vi "4155C Transfer.vi"(0 "VISA resource name in":refnum<visa-resource-name>="GPIB0::14::INSTR", 2 "Gate":T5={"Gate Start"=0.0, "Gate Stop"=2.0, "Gate Step (linear only)"=1.0, "Gate Compliance"=0.0001, "Gate PComp"=0.0, "Range mode"=0, "Range"=6} {"Range" max=11 scale=0.0..11.0; "Range mode" items=["Auto", "Limited", "Fixed"]; "Gate PComp" min=0.0 max=2.0 format="%^.2e"; "Gate Compliance" min=0.0 max=0.1 format="%^.2e"; "Gate Step (linear only)" min=-100.0 max=100.0 format="%^.4e"; "Gate Stop" min=-100.0 max=100.0 format="%^.4e"; "Gate Start" min=-100.0 max=100.0 format="%^.4e"}, 3 "Drain":T6={"Drain Start"=0.0, "Drain Stop"=2.0, "Drain Compliance"=0.0001, "Drain Step"=1.0, "Drain PComp"=0.0, "Range mode"=0, "Range"=6} {"Range" max=11 scale=0.0..11.0; "Range mode" items=["Auto", "Limited", "Fixed"]; "Drain PComp" min=0.0 max=2.0 format="%^.2e"; "Drain Step" min=-100.0 max=100.0 format="%^.4e"; "Drain Compliance" min=0.0 max=0.1 format="%^.2e"; "Drain Stop" min=-100.0 max=100.0 format="%^.4e"; "Drain Start" min=-100.0 max=100.0 format="%^.4e"}, 5 "Timings":T4={"integration time"=0, "Short/Long integration time"=0.00064, "hold time (sec)"=0.0, "delay time (sec)"=0.0, "Step Time (0 disables)"=0.0, "sweep method"=0, "Pulse period"=0.005, "Base voltage"=0.0, "Pulse width"=0.0005} {"Pulse width" min=0.0005 max=0.1 step=0.0001 format="%.4f"; "Base voltage" min=-100.0 max=100.0 format="%^.4e"; "Pulse period" min=0.005 max=1.0 step=0.0001 format="%.4f"; "sweep method" items=["Continuous", "Pulsed"]; "Step Time (0 disables)" min=0.0 format="%.2f"; "delay time (sec)" min=0.0 format="%.4f"; "hold time (sec)" min=0.0 format="%.4f"; "Short/Long integration time" min=0.0 format="%^.0e"; "integration time" scale=0.0..2.0}, 6 "error in (no error)":errorcluster, 7 "SMU4":cluster{"on/off":bool, "Voltage":dbl} {"Voltage" min=-100.0 max=100.0 format="%.2f"}, 10 "sweep mode":u16(ring) items=["Single", "Double"], 12 "Panel Controls":T3={"Emergency Stop"=refnum, "TransGraph Max"=1e-05, "Text/Graph (text=false)"=FALSE, "TransGraph Min"=1e-11} {"TransGraph Min" format="%.2e"; "TransGraph Max" format="%.2e"}, 13 "Standby":T1) -> (16 "VG":dbl[](array[numeric]) format="%.2f", 17 "Outparams":T2={"V2 Start"=0.0, "V2 Step"=0.0, "Number of points"=1} {"V2 Step" format="%.2f"; "V2 Start" format="%^.4e"}, 20 "VISA Resource Name out":refnum<visa-resource-name>, 22 "IS":dbl[](array[numeric]) format="%.2f", 23 "ID":dbl[](array[numeric]) format="%.2f", 25 "IG":dbl[](array[numeric]) format="%.2f", 26 "error out":errorcluster, 27 "SMU4":dbl[](array[numeric]) format="%.2f")   [LabVIEW 2016]
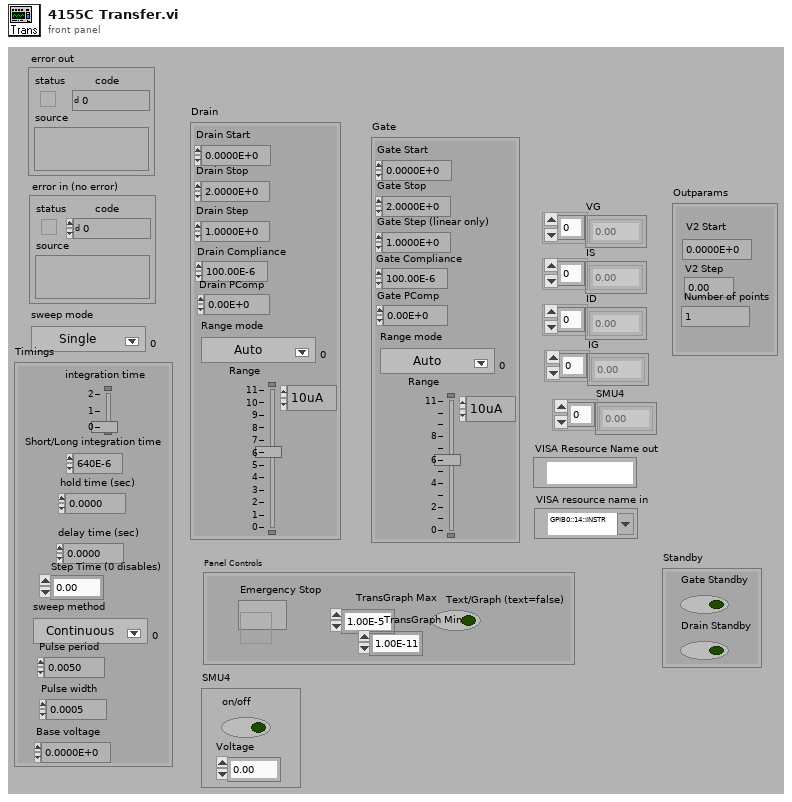
[diagram p1: front panel]
types:
  T1 = cluster{"Gate Standby":bool, "Drain Standby":bool}
  T2 = cluster{"V2 Start":dbl, "V2 Step":dbl, "Number of points":i32}
  T3 = cluster{"Emergency Stop":refnum<vi>, "TransGraph Max":dbl, "Text/Graph (text=false)":bool, "TransGraph Min":dbl}
  T4 = cluster{"integration time":u32, "Short/Long integration time":dbl, "hold time (sec)":dbl, "delay time (sec)":dbl, "Step Time (0 disables)":dbl, "sweep method":u16, "Pulse period":dbl, "Base voltage":dbl, "Pulse width":dbl}
  T5 = cluster{"Gate Start":dbl, "Gate Stop":dbl, "Gate Step (linear only)":dbl, "Gate Compliance":dbl, "Gate PComp":dbl, "Range mode":u16, "Range":u8}
  T6 = cluster{"Drain Start":dbl, "Drain Stop":dbl, "Drain Compliance":dbl, "Drain Step":dbl, "Drain PComp":dbl, "Range mode":u16, "Range":u8}
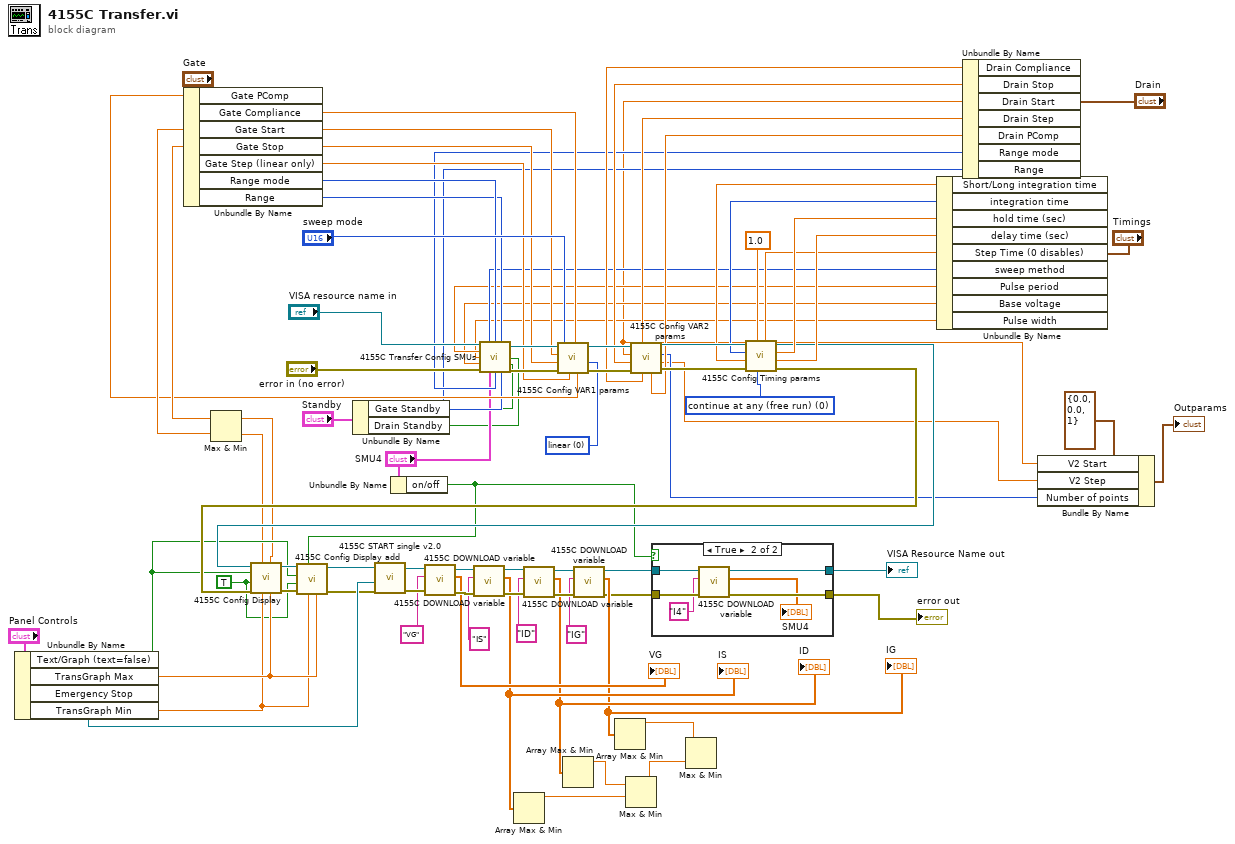
[diagram p0: block diagram]
diagram:
  w5 = TRUE ("Logarithmic")
  w69 = u8 0 items=["continue at any (free run)", "stop at any abnorm", "stop at compliance"] ("stop condition (free run:0)")
  w66 = u16 0 items=["linear", "log 10", "log 25", "log 50"] ("sweep spacing (linear: 0)")
  n1 = Unbundle By Name("Panel Controls") -> ("Text/Graph (text=false)"=w4:bool, "TransGraph Max"=w7:dbl, "Emergency Stop"=w36:refnum<vi>, "TransGraph Min"=w6:dbl)
  n2 = Unbundle By Name("Gate") -> ("Gate PComp"=w34:dbl, "Gate Compliance"=w55:dbl, "Gate Start"=w38:dbl, "Gate Stop"=w37:dbl, "Gate Step (linear only)"=w54:dbl, "Range mode"=w32:u16, "Range"=w31:u8)
  n3 = Max & Min(x=w37, y=w38) -> (max(x,y)=w1:dbl, min(x,y)=w2:dbl)
  n4 = Unbundle By Name("Standby") -> ("Gate Standby"=w13:bool, "Drain Standby"=w12:bool)
  n5 = Unbundle By Name("SMU4") -> ("on/off"=w3:bool)
  n6 = Unbundle By Name("Timings") -> ("Short/Long integration time"=w71:dbl, "integration time"=w49:u32, "hold time (sec)"=w50:dbl, "delay time (sec)"=w51:dbl, "Step Time (0 disables)"=w48:dbl, "sweep method"=w28:u16, "Pulse period"=w27:dbl, "Base voltage"=w25:dbl, "Pulse width"=w26:dbl)
  n7 = Unbundle By Name("Drain") -> ("Drain Compliance"=w58:dbl, "Drain Stop"=w57:dbl, "Drain Start"=w20:dbl, "Drain Step"=w56:dbl, "Drain PComp"=w33:dbl, "Range mode"=w30:u16, "Range"=w29:u8)
  n8 = call "4155C Transfer Config SMUs.vi"("VISA resource name in"="VISA resource name in", "sweep method"=w28, "Gate mode"=w32, "Gate Range"=w31, "Pulse period"=w27, "Pulse width"=w26, "Drain Standby"=w12, "Base voltage"=w25, "Gate Standby"=w13, "error in (no error)"="error in (no error)", "SMU4"="SMU4", "Source/drain mode"=w30, "Source/drain Range"=w29) -> ("VISA Resource Name out"=w64:refnum<visa-resource-name>, "error out"=w63:errorcluster)  [unwired: 1 in]
  n9 = call "4155C Config VAR1 params.vi"("sweep spacing (linear: 0)"=w66, "power compliance (0 = OFF)"=w34, "compliance"=w55, "step (linear only)"=w54, "sweep mode"="sweep mode", "error in (no error)"=w63, "stop"=w37, "start"=w38, "VISA session"=w64) -> ("error out"=w67:errorcluster, "dup VISA resource name"=w68:refnum<visa-resource-name>)  [unwired: 1 out]
  n10 = call "4155C Config VAR2 params.vi"("power compliance (0 = OFF)"=w33, "compliance"=w58, "step"=w56, "error in (no error)"=w67, "stop"=w57, "start"=w20, "VISA session"=w68) -> ("error out"=w72:errorcluster, "Corrected Step"=w21:dbl, "Number of points"=w22:i32, "dup VISA resource name"=w73:refnum<visa-resource-name>)  [unwired: 1 in]
  n11 = call "4155C Config Timing params.vi"("delay time (sec)"=w51, "hold time (sec)"=w50, "Step Time (0 disables)"=w48, "stop condition (free run:0)"=w69, "wait time parameter"=1.0, "error in (no error)"=w72, "Short/Long integration time"=w71, "integration time"=w49, "VISA session"=w73) -> ("error out"=w40:errorcluster, "dup VISA resource name"=w39:refnum<visa-resource-name>)  [unwired: 1 in]
  n12 = call "4155C Config Display.vi"("Ymax"=w7, "Var1 Stop"=w1, "Ymin"=w6, "Var1 Start"=w2, "error in (no error)"=w40, "Logarithmic"=w5, "SPA Display"=w4, "VISA session"=w39) -> ("error out"=w8:errorcluster, "dup VISA resource name"=w11:refnum<visa-resource-name>)  [unwired: 2 in]
  n13 = call "4155C Config Display add.vi"("Ymax"=w7, "Ymin"=w6, "SMU4"=w3, "error in (no error)"=w8, "Logarithmic"=w5, "SPA Display"=w4, "VISA session"=w11) -> ("error out"=w9:errorcluster, "dup VISA resource name"=w10:refnum<visa-resource-name>)  [unwired: 3 in]
  n14 = call "4155C START single v2.0.vi"("error in (no error)"=w9, "Emergency Stop"=w36, "VISA resource name in"=w10) -> ("error out"=w84:errorcluster, "VISA Resource Name out"=w85:refnum<visa-resource-name>)  [unwired: 3 in]
  n15 = call "4155C DOWNLOAD variable.vi"("error in (no error)"=w84, "Variable name"="VG", "VISA resource name in"=w85) -> ("error out"=w82:errorcluster, "Output data"=→"VG":dbl[], "VISA Resource Name out"=w81:refnum<visa-resource-name>)  [unwired: 2 in]
  n16 = call "4155C DOWNLOAD variable.vi"("error in (no error)"=w82, "Variable name"="IS", "VISA resource name in"=w81) -> ("error out"=w78:errorcluster, "Output data"=w47:dbl[], "VISA Resource Name out"=w79:refnum<visa-resource-name>)  [unwired: 2 in]
  "IS" <- w47
  n17 = Array Max & Min(array=w47) -> (max value=w44:dbl)  [unwired: 3 out]
  n18 = call "4155C DOWNLOAD variable.vi"("error in (no error)"=w78, "Variable name"="ID", "VISA resource name in"=w79) -> ("error out"=w77:errorcluster, "Output data"=w46:dbl[], "VISA Resource Name out"=w76:refnum<visa-resource-name>)  [unwired: 2 in]
  "ID" <- w46
  n19 = Array Max & Min(array=w46) -> (max value=w43:dbl)  [unwired: 3 out]
  n20 = call "4155C DOWNLOAD variable.vi"("error in (no error)"=w77, "Variable name"="IG", "VISA resource name in"=w76) -> ("error out"=w19:errorcluster, "Output data"=w45:dbl[], "VISA Resource Name out"=w18:refnum<visa-resource-name>)  [unwired: 2 in]
  "IG" <- w45
  n21 = Array Max & Min(array=w45) -> (max value=w42:dbl)  [unwired: 3 out]
  n22 = Max & Min(x=w43, y=w44) -> (max(x,y)=w41:dbl)  [unwired: 1 out]
  n23 = case shown="True" w3 {
    tunnel: w18 -> [w87 w93]
    tunnel: [w87 w90] -> w16
    tunnel: [w86 w91] -> w17
    tunnel: w19 -> [w86 w92]
    frame False {
    }
    frame True {
      n24 = call "4155C DOWNLOAD variable.vi"("error in (no error)"=w92, "Variable name"="I4", "VISA resource name in"=w93) -> ("error out"=w91:errorcluster, "Output data"=→"SMU4":dbl[], "VISA Resource Name out"=w90:refnum<visa-resource-name>)  [unwired: 2 in]
    }
  }
  "error out" <- w17
  "VISA Resource Name out" <- w16
  n25 = Max & Min(x=w42, y=w41) -> ()  [unwired: 2 out]
  n26 = Bundle By Name(cluster=T2 {"V2 Start"=0.0, "V2 Step"=0.0, "Number of points"=1} ("Outparams"), "V2 Start"=w20, "V2 Step"=w21, "Number of points"=w22) -> (→"Outparams":T2)
